vi "Create.vi"(10 "Node Info":T1) -> (3 "NodeInfoValue out":refnum<class "NodeInfoValue.lvclass">)   [LabVIEW 2020, in "Vecto.lvlib" / "NodeInfoValue.lvclass"]
uses:
  NodeInfoValue.lvclass
  Node Info.ctl
  Task Info.ctl
  NodeInfoValue.lvclass/NodeInfoValue.ctl
  Vecto.lvlib
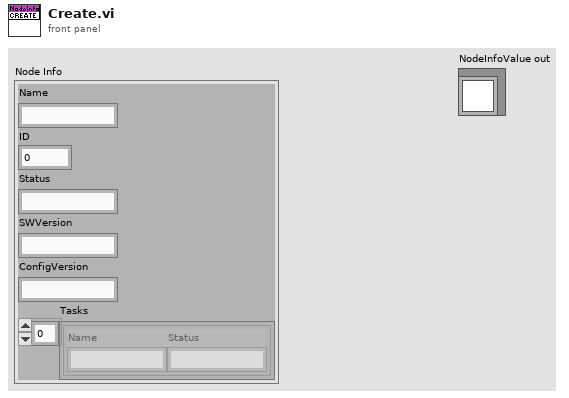
[diagram p1: front panel]
types:
  T1 = typedef "Vecto.lvlib/Node Info.ctl" = cluster{"Name":string, "ID":i32, "Status":string, "SWVersion":string, "ConfigVersion":string, "Tasks":T2[]}
  T2 = typedef "Vecto.lvlib/Task Info.ctl" = cluster{"Name":string, "Status":string}
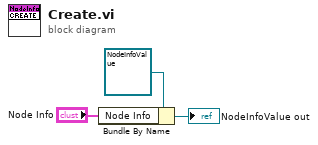
[diagram p0: block diagram]
diagram:
  n1 = Bundle By Name(cluster=refnum<class "NodeInfoValue.lvclass"> refnum ("NodeInfoValue in"), "Node Info"="Node Info") -> (→"NodeInfoValue out":refnum<class "NodeInfoValue.lvclass">)
